vi "OverWriteManualShiftValues.vi"(6 "AutoCenter":bool, 8 "Shift Beac Val":dbl, 9 "Shift Beac Ref":refnum<vi>, 10 "Shift Cal Val":dbl, 11 "Shift Cal Ref":refnum<vi>) -> ()   [LabVIEW 2018]
uses:
  Controls/Clusts/FreqShift.ctl
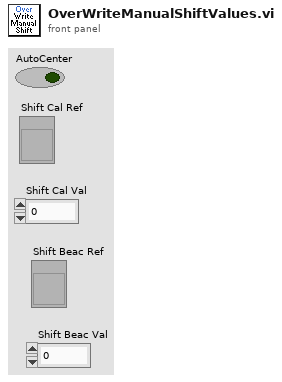
[diagram p1: front panel]
types:
  T1 = typedef "FreqShift.ctl" = cluster{"Fine":dbl, "Coarse_":dbl}
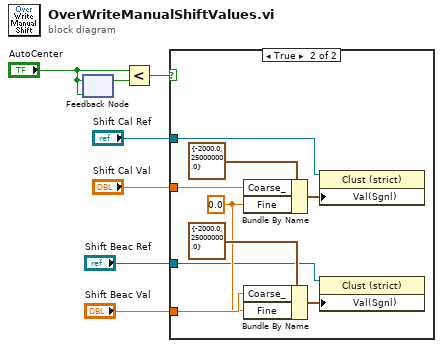
[diagram p0: block diagram]
diagram:
  n1 = feedback #1("AutoCenter") -> (w3:bool)
  n2 = feedback-in #1("AutoCenter") -> ()
  n3 = Less?(x="AutoCenter", y=w3) -> (x < y?=w4:bool)
  n4 = case shown="True" w4 {
    tunnel: "Shift Beac Val" -> [_ w16]
    tunnel: "Shift Cal Val" -> [_ w13]
    tunnel: "Shift Cal Ref" -> [_ w9]
    tunnel: "Shift Beac Ref" -> [_ w8]
    frame False {
    }
    frame True {
      w12 = 0.0 ("Fine")
      n5 = Bundle By Name(cluster=T1 {"Fine"=-2000.0, "Coarse_"=25000000.0} ("Shift Cal"), "Coarse_"=w13, "Fine"=w12) -> (w10:T1)
      n6 = Bundle By Name(cluster=T1 {"Fine"=-2000.0, "Coarse_"=25000000.0} ("Shift Cal"), "Coarse_"=w16, "Fine"=w12) -> (w11:T1)
      n7 = property class="Clust (strict)"(reference=w9, "Val(Sgnl)"=w10) -> ()  [unwired: 1 in, 2 out]
      n8 = property class="Clust (strict)"(reference=w8, "Val(Sgnl)"=w11) -> ()  [unwired: 1 in, 2 out]
    }
  }
